vi "LVPortGetNamepathValue.vi"(8 "error in":errorcluster, 9 "Namepath Data in":T1, 10 "Object ID":i32, 11 "pID":string) -> (0 "error out":errorcluster, 2 "Invalid Indexing or errored value":bool, 3 "Namepath Data out":T1)   [LabVIEW 2017]
uses:
  Common/ObjectMap/LVPortObjectMapNamepathData.ctl
  Common/ObjectMap/LVPortObjectMapDataTypeEnum.ctl
  Common/ObjectMap/LVPortObjectMapContainerTypeEnum.ctl
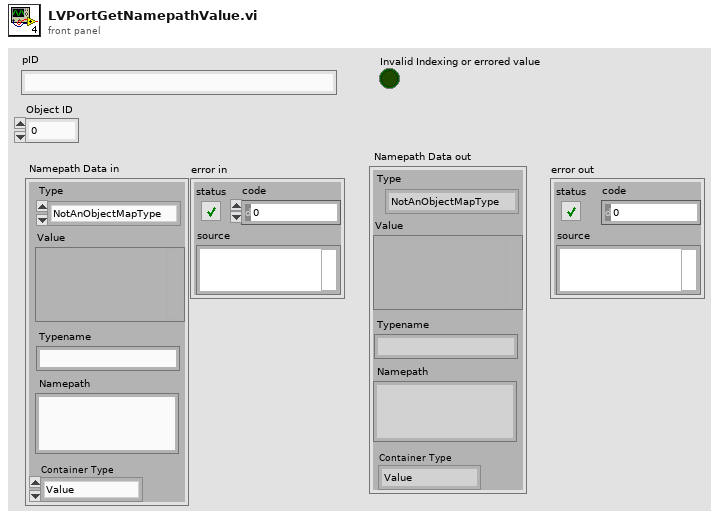
[diagram p1: front panel]
types:
  T1 = typedef "LVPortObjectMapNamepathData.ctl" = cluster{"Type":T2, "Value":variant, "Namepath":string, "Typename":string, "Container Type":T3}
  T2 = typedef "LVPortObjectMapDataTypeEnum.ctl" = enum16{"NotAnObjectMapType", "Real", "Complex", "String", "Boolean"}
  T3 = typedef "LVPortObjectMapContainerTypeEnum.ctl" = enum16{"Value", "Array", "Waveform"}
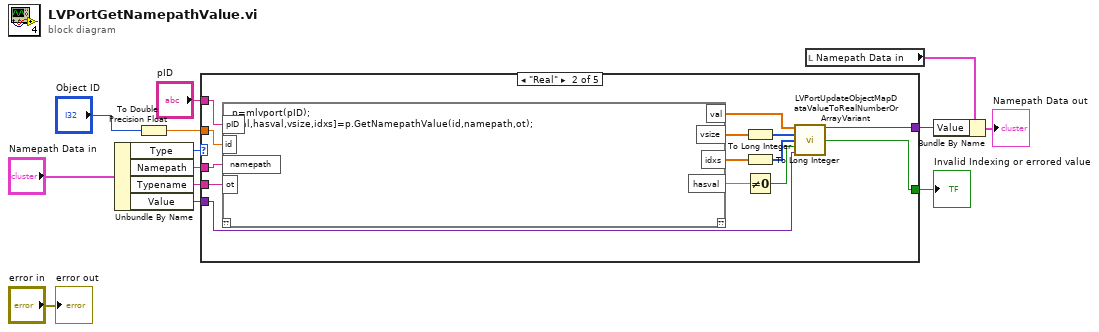
[diagram p0: block diagram]
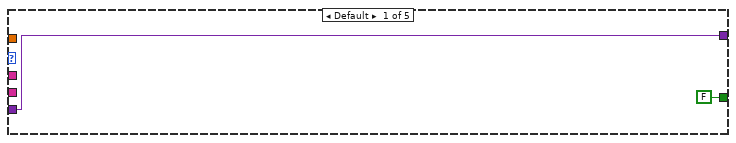
[diagram p2: hidden frame]
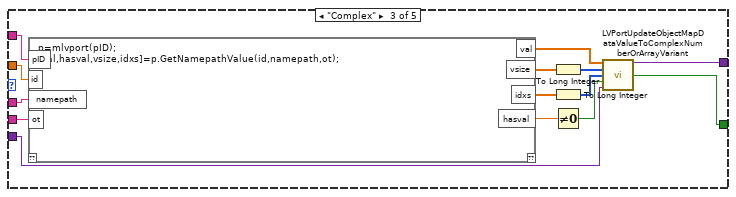
[diagram p3: hidden frame]
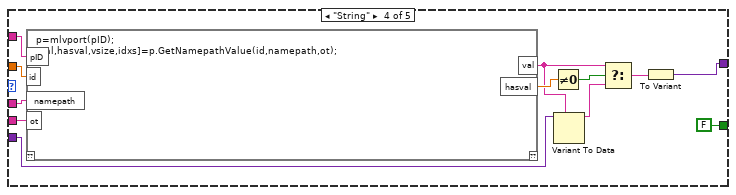
[diagram p4: hidden frame]
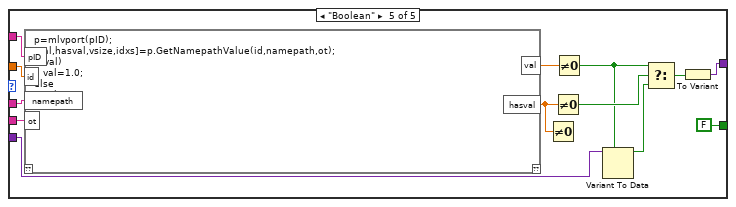
[diagram p5: hidden frame]
diagram:
  n1 = Unbundle By Name("Namepath Data in") -> ("Type"=w11:T2, "Namepath"=w6:string, "Typename"=w10:string, "Value"=w3:variant)
  n2 = To Double Precision Float(number="Object ID") -> (double precision float=w4:dbl)
  n3 = case shown="\"Real\"" w11 {
    tunnel: [w15 w27 w41 w48 w60] -> w8
    tunnel: "pID" -> [_ w29 w43 w55 w67]
    tunnel: w4 -> [_ w25 w39 w47 w59]
    tunnel: w10 -> [_ w23 w37 w45 w57]
    tunnel: w6 -> [_ w24 w38 w46 w58]
    tunnel: w3 -> [w15 w17 w31 w54 w63]
    tunnel: [FALSE ("Invalid Indexing or errored value") w16 w30 FALSE ("Invalid Indexing or errored value") FALSE ("Invalid Indexing or errored value")] -> w1
    frame Default {
    }
    frame "Real" {
      n4 = script code="p=mlvport(pID);\n[val,hasval,vsize,idxs]=p.GetNamepathValue(id,namepath,ot);"("pID"=w29, "id"=w25, "ot"=w23, "namepath"=w24) -> ("val"=w28:dbl[], "vsize"=w19:dbl[], "hasval"=w26:dbl, "idxs"=w21:dbl[])  [unwired: 1 in, 1 out]
      n5 = To Long Integer(number=w19) -> (32bit integer=w18:i32[])
      n6 = To Long Integer(number=w21) -> (32bit integer=w20:i32[])
      n7 = Not Equal To 0?(x=w26) -> (x != 0?=w22:bool)
      n8 = call "LVPortUpdateObjectMapDataValueToRealNumberOrArrayVariant.vi"("UpdateData"=w28, "Sizes"=w18, "UpdateAt"=w20, "Has Value"=w22, "SourceValue"=w17) -> ("Value"=w27:variant, "Invalid Indexing or errored value"=w16:bool)  [unwired: 9 in]
    }
    frame "Complex" {
      n9 = script code="p=mlvport(pID);\n[val,hasval,vsize,idxs]=p.GetNamepathValue(id,namepath,ot);"("pID"=w43, "id"=w39, "ot"=w37, "namepath"=w38) -> ("val"=w42:cdb[], "vsize"=w33:dbl[], "hasval"=w40:dbl, "idxs"=w35:dbl[])  [unwired: 1 in, 1 out]
      n10 = To Long Integer(number=w33) -> (32bit integer=w32:i32[])
      n11 = To Long Integer(number=w35) -> (32bit integer=w34:i32[])
      n12 = Not Equal To 0?(x=w40) -> (x != 0?=w36:bool)
      n13 = call "LVPortUpdateObjectMapDataValueToComplexNumberOrArrayVariant.vi"("UpdatedData"=w42, "Sizes"=w32, "UpdateAt"=w34, "Has Value"=w36, "SourceValue"=w31) -> ("Value"=w41:variant, "Invalid Indexing or errored value"=w30:bool)  [unwired: 9 in]
    }
    frame "String" {
      n14 = script code="p=mlvport(pID);\n[val,hasval,vsize,idxs]=p.GetNamepathValue(id,namepath,ot);"("pID"=w55, "id"=w47, "namepath"=w46, "ot"=w45) -> ("val"=w50:string, "hasval"=w53:dbl)  [unwired: 1 in, 1 out]
      n15 = Not Equal To 0?(x=w53) -> (x != 0?=w52:bool)
      n16 = Variant To Data(type=w50, Variant=w54) -> (data=w51:string)  [unwired: 1 in, 1 out]
      n17 = Select(t=w50, s=w52, f=w51) -> (s? t:f=w49:string)
      n18 = To Variant(anything=w49) -> (Variant=w48:variant)
    }
    frame "Boolean" {
      n19 = script code="p=mlvport(pID);\n[val,hasval,vsize,idxs]=p.GetNamepathValue(id,namepath,ot);\nif(val)\n   val=1.0;\nelse\n   val=0.0;\nend"("pID"=w67, "id"=w59, "namepath"=w58, "ot"=w57) -> ("val"=w68:dbl, "hasval"=w62:dbl)  [unwired: 1 in, 1 out]
      n20 = Not Equal To 0?(x=w62) -> ()  [unwired: 1 out]
      n21 = Not Equal To 0?(x=w62) -> (x != 0?=w66:bool)
      n22 = Not Equal To 0?(x=w68) -> (x != 0?=w61:bool)
      n23 = Variant To Data(type=w61, Variant=w63) -> (data=w65:bool)  [unwired: 1 in, 1 out]
      n24 = Select(t=w61, s=w66, f=w65) -> (s? t:f=w64:bool)
      n25 = To Variant(anything=w64) -> (Variant=w60:variant)
    }
  }
  "Invalid Indexing or errored value" <- w1
  n26 = local read "Namepath Data in"() -> (w9:T1)
  n27 = Bundle By Name(cluster=w9, "Value"=w8) -> (→"Namepath Data out":T1)
  "error out" <- "error in"
